vi "Periodic Tasks.vi"() -> ()   [LabVIEW 2012]
doc: "This VI runs in parallel to other tasks. It can contain as many user-defined periodic loops as you need. These can carry out PID or other sorts of timed response."
uses:
  <vilib>/Rock Robotics/SystemInterfaces/Utilities/FPGA_UtilitiesLED Source.ctl
  <vilib>/Rock Robotics/SystemInterfaces/Utilities/FPGA_UtilitiesLED State.ctl
  Robot Global Data.vi
panel:
  in  "Shoot Deadband":dbl=0.05
  out "Angular Rate":dbl
  out "Angle":dbl
  out "Rate":dbl
  out "Direction":bool
  out "Distance":dbl
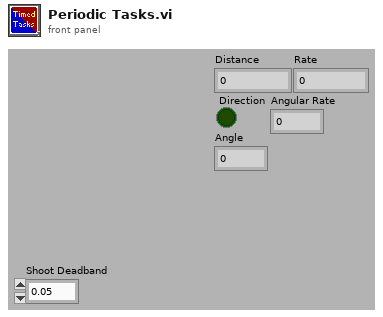
[diagram p1: front panel]
types:
  T1 = typedef "FPGA_UtilitiesLED State.ctl" = enum16{"Off", "On", "Toggle"}
  T2 = typedef "FPGA_UtilitiesLED Source.ctl" = enum16{"User LED", "FPGA LED"}
  T3 = cluster{"ClimbManualExt":dbl, "ClimbManualDep":dbl, "ClimbRetEnable":bool, "ClimbPOTDep":dbl, "ClimbConst":cluster{"ClimbConstDep":dbl, "ClimbConstFold":dbl, "ClimbConstExt":dbl, "ClimbConstRet":dbl}, "ClimbPOTExt":dbl, "ClimbExtEnable":bool, "ClimbLimit":bool, "ClimbFoldEnable":bool, "ClimbDepEnable":bool, "ClimbCase":dbl}
  T4 = cluster{"ShootTrackEnable":bool, "ShootStartWheels":bool, "ShootIndexerEnable":bool, "ShootCase":dbl, "ShootPOTElev":dbl, "ShootManualElev":dbl, "IndexerSpeed":dbl, "Default Wheel Speed":dbl, "Deadband":dbl, "ShootTargetInfo":cluster{"X Coord":dbl, "Y Coord":dbl, "Distance":dbl}, "ShootConstElev":cluster{"1":dbl, "2":dbl, "3":dbl, "4":dbl, "Ground":dbl}, "ShootRollerSpd":dbl, "ShootFlipperPE":bool, "ShootConstFlipper":cluster{"Down":dbl, "Up":dbl}}
  T5 = typedef "WPI_GyroDevRef.ctl" = cluster{"DevStatus":errorcluster, "Analog Module":T6, "Analog Channel":T7, "Offset":dbl, "Gain (VoltsPerDegree/Second)":dbl}
  T6 = typedef "FPGA_TypedefAnalogModule.ctl" = enum16{"Analog Module 1", "Analog Module 2"}
  T7 = typedef "FPGA_AIChannel.ctl" = enum8{"AI 1", "AI 2", "AI 3", "AI 4", "AI 5", "AI 6", "AI 7", "AI 8", "Invalid"}
  T8 = typedef "WPI_EncoderDevRef.ctl" = cluster{"DevStatus":errorcluster, "EncoderIndex":T9, "CounterIndex":T10, "DistancePerCount":dbl, "Decoding Type":T11}
  T9 = typedef "FPGA_EncoderIdx.ctl" = enum8{"Enc 0", "Enc 1", "Enc 2", "Enc 3", "Invalid"}
  T10 = typedef "FPGA_CounterCtrSystemIndex.ctl" = enum8{"Ctr 0", "Ctr 1", "Ctr 2", "Ctr 3", "Ctr 4", "Ctr 5", "Ctr 6", "Ctr 7", "Invalid"}
  T11 = typedef "WPI_EncoderType.ctl" = enum16{"1x", "2x", "4x"}
  T12 = typedef "WPI_DigitalInputDevRef.ctl" = cluster{"DevStatus":errorcluster, "DIO Channel":T13, "Digital Module":T14}
  T13 = typedef "FPGA_DIOChannel.ctl" = enum8{"DIO 1", "DIO 2", "DIO 3", "DIO 4", "DIO 5", "DIO 6", "DIO 7", "DIO 8", "DIO 9", "DIO 10", "DIO 11", "DIO 12", "DIO 13", "DIO 14", "Invalid"}
  T14 = typedef "FPGA_TypedefDigitalModule.ctl" = enum16{"Digital Module 1", "Digital Module 2"}
  T15 = typedef "WPI_AnalogChannelDevRef.ctl" = cluster{"DevStatus":errorcluster, "Analog Module":T6, "Analog Channel":T7}
  T16 = cluster{"Ground":dbl, "1":dbl, "2":dbl, "3":dbl, "4":dbl}
  T17 = cluster{"ClimbConstDep":dbl, "ClimbConstFold":dbl, "ClimbConstExt":dbl, "ClimbConstRet":dbl}
  T18 = cluster{"ClimbOutDep":dbl, "ClimbOutExt":dbl, "ClimbOutCase":i32}
  T19 = cluster{"ShootOutIndexer":dbl, "ShootOutElev":dbl, "ShootOutCase":dbl, "ShootOutWheelF":dbl, "ShootOutRollers":dbl, "ShootOutFlipper":dbl}
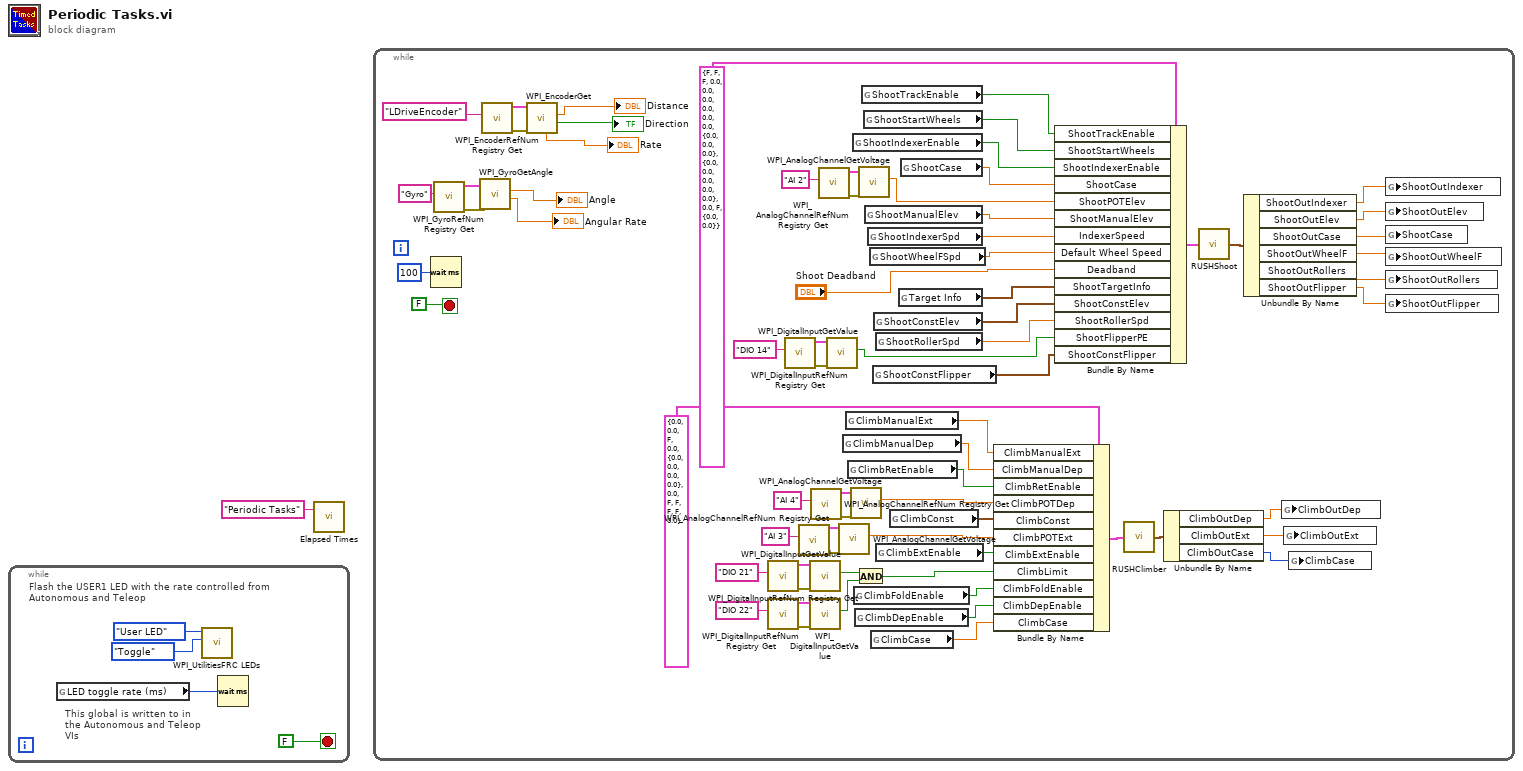
[diagram p0: block diagram]
diagram:
  n1 = while {
    stop <- FALSE stop-if-true
    # "This global is written to in the Autonomous and Teleop VIs"
    # "Flash the USER1 LED with the rate controlled from Autonomous and Teleop"
    n2 = global read "Robot Global Data.vi" "LED toggle rate (ms)"() -> (w2:u32)
    n3 = call <vilib>:"WPI_UtilitiesFRC LEDs.vi"("State"=FPGA_UtilitiesLED_State."Toggle", "LED Type"=FPGA_UtilitiesLED_Source."User LED") -> ()  [unwired: 1 in, 9 out]
    n4 = Wait (ms)(milliseconds to wait=w2) -> ()  [unwired: 1 out]
  }
  n5 = call "Elapsed Times.vi"("Call Name"="Periodic Tasks") -> ()  [unwired: 2 in, 1 out]
  n6 = while {
    stop <- FALSE stop-if-true
    n7 = Wait (ms)(milliseconds to wait=u32 100) -> ()  [unwired: 1 out]
    n8 = call <vilib>:"WPI_GyroRefNum Registry Get.vi"("refnum name"="Gyro") -> ("error out"=w74:errorcluster, "GyroDevRef"=w73:T5)  [unwired: 9 in]
    n9 = call <vilib>:"WPI_GyroGetAngle.vi"("error in (no error)"=w74, "GyroDevRef"=w73) -> ("Angular Rate"=→"Angular Rate":dbl, "Angle"=→"Angle":dbl)  [unwired: 6 in, 2 out]
    n10 = call <vilib>:"WPI_EncoderRefNum Registry Get.vi"("refnum name"="LDriveEncoder") -> ("error out"=w76:errorcluster, "EncoderDevRef"=w75:T8)  [unwired: 9 in]
    n11 = call <vilib>:"WPI_EncoderGet.vi"("error in (no error)"=w76, "EncoderDevRef"=w75) -> ("Direction"=→"Direction":bool, "Distance"=→"Distance":dbl, "Rate"=→"Rate":dbl)  [unwired: 4 in, 3 out]
    n12 = call <vilib>:"WPI_DigitalInputRefNum Registry Get.vi"("refnum name"="DIO 21") -> ("error out"=w31:errorcluster, "DigitalInputDevRef"=w32:T12)  [unwired: 9 in]
    n13 = call <vilib>:"WPI_DigitalInputRefNum Registry Get.vi"("refnum name"="DIO 22") -> ("error out"=w30:errorcluster, "DigitalInputDevRef"=w29:T12)  [unwired: 9 in]
    n14 = call <vilib>:"WPI_DigitalInputRefNum Registry Get.vi"("refnum name"="DIO 14") -> ("error out"=w41:errorcluster, "DigitalInputDevRef"=w40:T12)  [unwired: 9 in]
    n15 = call <vilib>:"WPI_AnalogChannelRefNum Registry Get.vi"("refnum name"="AI 3") -> ("error out"=w19:errorcluster, "AIDeviceRef"=w18:T15)  [unwired: 9 in]
    n16 = call <vilib>:"WPI_DigitalInputGetValue.vi"("error in (no error)"=w31, "DigitalInputDevRef"=w32) -> ("Value"=w26:bool)  [unwired: 7 in, 2 out]
    n17 = call <vilib>:"WPI_DigitalInputGetValue.vi"("error in (no error)"=w30, "DigitalInputDevRef"=w29) -> ("Value"=w27:bool)  [unwired: 7 in, 2 out]
    n18 = call <vilib>:"WPI_AnalogChannelRefNum Registry Get.vi"("refnum name"="AI 4") -> ("error out"=w24:errorcluster, "AIDeviceRef"=w22:T15)  [unwired: 9 in]
    n19 = call <vilib>:"WPI_AnalogChannelRefNum Registry Get.vi"("refnum name"="AI 2") -> ("error out"=w44:errorcluster, "AIDeviceRef"=w43:T15)  [unwired: 9 in]
    n20 = call <vilib>:"WPI_DigitalInputGetValue.vi"("error in (no error)"=w41, "DigitalInputDevRef"=w40) -> ("Value"=w38:bool)  [unwired: 7 in, 2 out]
    n21 = call <vilib>:"WPI_AnalogChannelGetVoltage.vi"("error in (no error)"=w19, "AIDeviceRef"=w18) -> ("Voltage"=w17:dbl)  [unwired: 7 in, 2 out]
    n22 = global read "Robot Global Data.vi" "ClimbManualDep"() -> (w15:dbl)
    n23 = global read "Robot Global Data.vi" "ClimbManualExt"() -> (w16:dbl)
    n24 = global read "Robot Global Data.vi" "ClimbRetEnable"() -> (w14:bool)
    n25 = call <vilib>:"WPI_AnalogChannelGetVoltage.vi"("error in (no error)"=w24, "AIDeviceRef"=w22) -> ("Voltage"=w21:dbl)  [unwired: 7 in, 2 out]
    n26 = global read "Robot Global Data.vi" "ShootIndexerEnable"() -> (w55:bool)
    n27 = global read "Robot Global Data.vi" "ClimbFoldEnable"() -> (w11:bool)
    n28 = global read "Robot Global Data.vi" "ClimbDepEnable"() -> (w10:bool)
    n29 = And(x=w26, y=w27) -> (x .and. y?=w25:bool)
    n30 = call <vilib>:"WPI_AnalogChannelGetVoltage.vi"("error in (no error)"=w44, "AIDeviceRef"=w43) -> ("Voltage"=w42:dbl)  [unwired: 7 in, 2 out]
    n31 = global read "Robot Global Data.vi" "ShootTrackEnable"() -> (w57:bool)
    n32 = global read "Robot Global Data.vi" "ShootStartWheels"() -> (w56:bool)
    n33 = global read "Robot Global Data.vi" "ShootManualElev"() -> (w54:dbl)
    n34 = global read "Robot Global Data.vi" "ShootIndexerSpd"() -> (w64:dbl)
    n35 = global read "Robot Global Data.vi" "ShootWheelFSpd"() -> (w63:dbl)
    n36 = global read "Robot Global Data.vi" "ClimbCase"() -> (w9:dbl)
    n37 = global read "Robot Global Data.vi" "ShootConstFlipper"() -> (w60:cluster{"Down":dbl, "Up":dbl})
    n38 = global read "Robot Global Data.vi" "ShootConstElev"() -> (w61:T16)
    n39 = global read "Robot Global Data.vi" "ShootRollerSpd"() -> (w53:dbl)
    n40 = global read "Robot Global Data.vi" "ClimbExtEnable"() -> (w12:bool)
    n41 = global read "Robot Global Data.vi" "ClimbConst"() -> (w13:T17)
    n42 = global read "Robot Global Data.vi" "Target Info"() -> (w62:cluster{"X":dbl, "Y":dbl, "Distance (ft)":dbl})
    n43 = global read "Robot Global Data.vi" "ShootCase"() -> (w65:dbl)
    n44 = Bundle By Name(cluster=T3 {"ClimbManualExt"=0.0, "ClimbManualDep"=0.0, "ClimbRetEnable"=FALSE, "ClimbPOTDep"=0.0, "ClimbConst"={"ClimbConstDep"=0.0, "ClimbConstFold"=0.0, "ClimbConstExt"=0.0, "ClimbConstRet"=0.0}, "ClimbPOTExt"=0.0, "ClimbExtEnable"=FALSE, "ClimbLimit"=FALSE, "ClimbFoldEnable"=FALSE, "ClimbDepEnable"=FALSE, "ClimbCase"=0.0} ("In Cluster 2"), "ClimbManualExt"=w16, "ClimbManualDep"=w15, "ClimbRetEnable"=w14, "ClimbPOTDep"=w21, "ClimbConst"=w13, "ClimbPOTExt"=w17, "ClimbExtEnable"=w12, "ClimbLimit"=w25, "ClimbFoldEnable"=w11, "ClimbDepEnable"=w10, "ClimbCase"=w9) -> (w35:T3)
    n45 = Bundle By Name(cluster=T4 {"ShootTrackEnable"=FALSE, "ShootStartWheels"=FALSE, "ShootIndexerEnable"=FALSE, "ShootCase"=0.0, "ShootPOTElev"=0.0, "ShootManualElev"=0.0, "IndexerSpeed"=0.0, "Default Wheel Speed"=0.0, "Deadband"=0.0, "ShootTargetInfo"={"X Coord"=0.0, "Y Coord"=0.0, "Distance"=0.0}, "ShootConstElev"={"1"=0.0, "2"=0.0, "3"=0.0, "4"=0.0, "Ground"=0.0}, "ShootRollerSpd"=0.0, "ShootFlipperPE"=FALSE, "ShootConstFlipper"={"Down"=0.0, "Up"=0.0}} ("In Cluster"), "ShootTrackEnable"=w57, "ShootStartWheels"=w56, "ShootIndexerEnable"=w55, "ShootCase"=w65, "ShootPOTElev"=w42, "ShootManualElev"=w54, "IndexerSpeed"=w64, "Default Wheel Speed"=w63, "Deadband"="Shoot Deadband", "ShootTargetInfo"=w62, "ShootConstElev"=w61, "ShootRollerSpd"=w53, "ShootFlipperPE"=w38, "ShootConstFlipper"=w60) -> (w58:T4)
    n46 = call "RUSHClimber.vi"("In Cluster"=w35) -> ("Out Cluster"=w34:T18)
    n47 = Unbundle By Name(w34) -> ("ClimbOutDep"=w6:dbl, "ClimbOutExt"=w7:dbl, "ClimbOutCase"=w8:i32)
    n48 = call "RUSHShoot.vi"("In Cluster"=w58) -> ("Out Cluster"=w52:T19)
    n49 = Unbundle By Name(w52) -> ("ShootOutIndexer"=w49:dbl, "ShootOutElev"=w50:dbl, "ShootOutCase"=w51:dbl, "ShootOutWheelF"=w48:dbl, "ShootOutRollers"=w47:dbl, "ShootOutFlipper"=w46:dbl)
    n50 = global write "Robot Global Data.vi" "ClimbOutDep"(w6) -> ()
    n51 = global write "Robot Global Data.vi" "ClimbOutExt"(w7) -> ()
    n52 = global write "Robot Global Data.vi" "ClimbCase"(w8) -> ()
    n53 = global write "Robot Global Data.vi" "ShootOutIndexer"(w49) -> ()
    n54 = global write "Robot Global Data.vi" "ShootOutElev"(w50) -> ()
    n55 = global write "Robot Global Data.vi" "ShootCase"(w51) -> ()
    n56 = global write "Robot Global Data.vi" "ShootOutWheelF"(w48) -> ()
    n57 = global write "Robot Global Data.vi" "ShootOutRollers"(w47) -> ()
    n58 = global write "Robot Global Data.vi" "ShootOutFlipper"(w46) -> ()
  }
